vi "SQLite Add Saving Goal Test.vi"(7 "Test DB Set Up Command":string, 8 "Error In (no error)":errorcluster, 11 "SQLite DB Operator In":refnum<class "SQLite DB Operator.lvclass">) -> (0 "Error Out":errorcluster, 3 "SQLite DB Operator Out":refnum<class "SQLite DB Operator.lvclass">)   [LabVIEW 2023]
uses:
  Clasess/SQLite DB Operator/SQLite DB Operator.lvclass
  Clasess/DB Records/Expenses Tracker Saving Goal/Public/Ctrls/Saving Goal.ctl
  Clasess/DB Records/Expenses Tracker Saving Goal/Expenses Tracker Saving Goal.lvclass
  H:/Desktop/LabVIEW/LabView Repo/Expenses-Tracker-DB-Operator/Interfaces/Expenses Tracker Record/Expenses Tracker Record.lvclass
  Clasess/DB Records/Expenses Tracker Transaction/Expenses Tracker Transaction.lvclass
  Support/Adding/Add Record Assert Error.vi
  Support/Adding/Add Record Assert Not Error.vi
  <vilib>/drjdpowell/SQLite Library/SQL Connection/Execute SQL (1D Cluster).vi
  <vilib>/addons/_JKI Toolkits/Caraya/classes/Test/Test.lvclass
  <vilib>/drjdpowell/SQLite Library/SQLite.lvlib
  H:/Desktop/LabVIEW/LabView Repo/Expenses-Tracker-DB-Operator/Clasess/DB Records/Expenses Tracker Saving Goal/Expenses Tracker Saving Goal.lvclass
  <vilib>/drjdpowell/SQLite Library/SQL Connection/Connection.lvclass
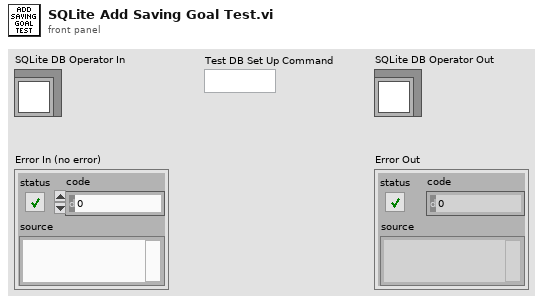
[diagram p1: front panel]
types:
  T1 = typedef "Expenses Tracker Saving Goal.lvclass/Saving Goal.ctl" = cluster{"ID":u32, "Name":string, "Current_value":dbl, "Target_value":dbl, "Date_of_entry":timestamp, "Due_date":timestamp, "Last_update":timestamp, "Description":string}
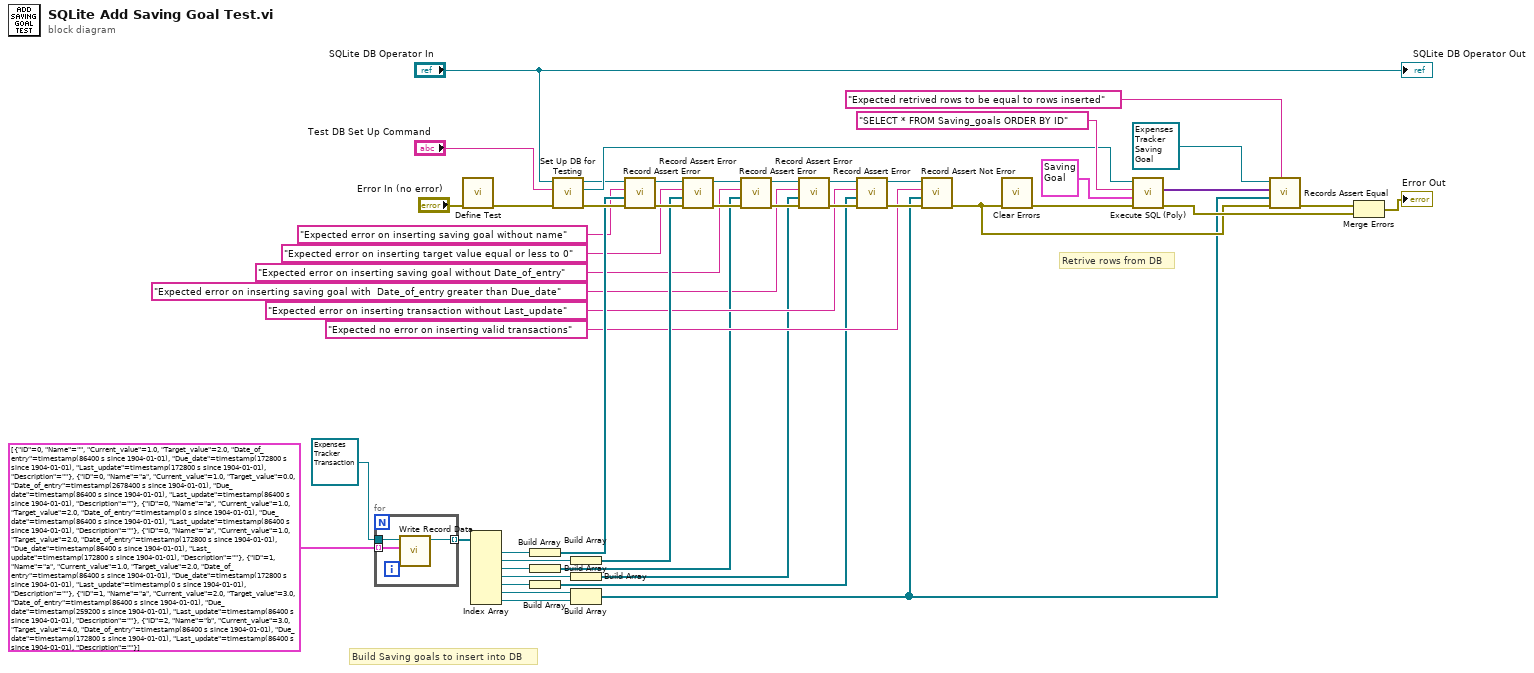
[diagram p0: block diagram]
diagram:
  (unwired) refnum<class "Expenses Tracker Transaction.lvclass"> refnum ("Expenses Tracker Category")
  # "Retrive rows from DB"
  # "Build Saving goals to insert into DB"
  n1 = for {
    tunnel: T1[] [{"ID"=0, "Name"="", "Current_value"=1.0, "Target_value"=2.0, "Date_of_entry"=timestamp(86400 s since 1904-01-01), "Due_date"=timestamp(172800 s since 1904-01-01), "Last_update"=timestamp(172800 s since 1904-01-01), "Description"=""}, {"ID"=0, "Name"="a", "Current_value"=1.0, "Target_value"=0.0, "Date_of_entry"=timestamp(2678400 s since 1904-01-01), "Due_date"=timestamp(86400 s since 1904-01-01), "Last_update"=timestamp(86400 s since 1904-01-01), "Description"=""}, {"ID"=0, "Name"="a", "Current_value"=1.0, "Target_value"=2.0, "Date_of_entry"=timestamp(0 s since 1904-01-01), "Due_date"=timestamp(86400 s since 1904-01-01), "Last_update"=timestamp(86400 s since 1904-01-01), "Description"=""}, {"ID"=0, "Name"="a", "Current_value"=1.0, "Target_value"=2.0, "Date_of_entry"=timestamp(172800 s since 1904-01-01), "Due_date"=timestamp(86400 s since 1904-01-01), "Last_update"=timestamp(172800 s since 1904-01-01), "Description"=""}, {"ID"=1, "Name"="a", "Current_value"=1.0, "Target_value"=2.0, "Date_of_entry"=timestamp(86400 s since 1904-01-01), "Due_date"=timestamp(172800 s since 1904-01-01), "Last_update"=timestamp(0 s since 1904-01-01), "Description"=""}, {"ID"=1, "Name"="a", "Current_value"=2.0, "Target_value"=3.0, "Date_of_entry"=timestamp(86400 s since 1904-01-01), "Due_date"=timestamp(259200 s since 1904-01-01), "Last_update"=timestamp(86400 s since 1904-01-01), "Description"=""}, {"ID"=2, "Name"="b", "Current_value"=3.0, "Target_value"=4.0, "Date_of_entry"=timestamp(86400 s since 1904-01-01), "Due_date"=timestamp(172800 s since 1904-01-01), "Last_update"=timestamp(86400 s since 1904-01-01), "Description"=""}] ("Array") -> [w52] mode=indexing
    tunnel: refnum<class "Expenses Tracker Saving Goal.lvclass"> refnum ("Expenses Tracker Category") -> [w50]
    tunnel: [w51] -> w47 mode=indexing
    n2 = call-dynamic "Write Record Data.vi"("Record"=w52, "Expenses Tracker Saving Goal In"=w50) -> ("Expenses Tracker Saving Goal Out"=w51:refnum<class "Expenses Tracker Saving Goal.lvclass">)  [unwired: 8 in, 1 out]
  }
  n3 = call <vilib>:"Define Test.vi"("error in (no error)"="Error In (no error)") -> ("error out"=w41:errorcluster)  [unwired: 9 in, 1 out]
  n4 = Index Array(array=w47) -> (element #1=w23:refnum<class "Expenses Tracker Saving Goal.lvclass">, element #2=w19:refnum<class "Expenses Tracker Saving Goal.lvclass">, element #3=w14:refnum<class "Expenses Tracker Saving Goal.lvclass">, element #4=w12:refnum<class "Expenses Tracker Saving Goal.lvclass">, element #5=w10:refnum<class "Expenses Tracker Saving Goal.lvclass">, element #6=w2:refnum<class "Expenses Tracker Saving Goal.lvclass">, element #7=w1:refnum<class "Expenses Tracker Saving Goal.lvclass">)  [unwired: 7 in]
  n5 = Build Array(w23) -> (w22:refnum<class "Expenses Tracker Saving Goal.lvclass">[])
  n6 = Build Array(w14) -> (w13:refnum<class "Expenses Tracker Saving Goal.lvclass">[])
  n7 = Build Array(w10) -> (w9:refnum<class "Expenses Tracker Saving Goal.lvclass">[])
  n8 = call "Set Up DB for Testing.vi"("Error In (no error)"=w41, "Test DB Set Up Command"="Test DB Set Up Command", "SQLite DB Operator In"="SQLite DB Operator In") -> ("Error Out"=w25:errorcluster, "SQLite Connection"=w44:refnum<class "Connection.lvclass">, "SQLite DB Operator Out"=w21:refnum<class "SQLite DB Operator.lvclass">)  [unwired: 6 in]
  n9 = Build Array(w19) -> (w18:refnum<class "Expenses Tracker Saving Goal.lvclass">[])
  n10 = Build Array(w12) -> (w11:refnum<class "Expenses Tracker Saving Goal.lvclass">[])
  n11 = Build Array(w2, w1) -> (w3:refnum<class "Expenses Tracker Saving Goal.lvclass">[])
  n12 = call-poly "Record Assert Error.vi"("Error In"=w25, "Records"=w22, "Assertion Label"="Expected error on inserting saving goal without name" ("Label (VI Title)"), "SQLite DB Operator In"=w21) -> ("Error Out"=w32:errorcluster, "SQLite DB Operator Out"=w33:refnum<class "SQLite DB Operator.lvclass">)  [unwired: 6 in]
  n13 = call-poly "Record Assert Error.vi"("Error In"=w32, "Records"=w18, "Assertion Label"="Expected error on inserting target value equal or less to 0" ("Label (VI Title)"), "SQLite DB Operator In"=w33) -> ("Error Out"=w30:errorcluster, "SQLite DB Operator Out"=w31:refnum<class "SQLite DB Operator.lvclass">)  [unwired: 6 in]
  n14 = call-poly "Record Assert Error.vi"("Error In"=w30, "Records"=w13, "Assertion Label"="Expected error on inserting saving goal without Date_of_entry" ("Label (VI Title)"), "SQLite DB Operator In"=w31) -> ("Error Out"=w35:errorcluster, "SQLite DB Operator Out"=w34:refnum<class "SQLite DB Operator.lvclass">)  [unwired: 6 in]
  n15 = call-poly "Record Assert Error.vi"("Error In"=w35, "Records"=w11, "Assertion Label"="Expected error on inserting saving goal with  Date_of_entry greater than Due_date" ("Label (VI Title)"), "SQLite DB Operator In"=w34) -> ("Error Out"=w28:errorcluster, "SQLite DB Operator Out"=w29:refnum<class "SQLite DB Operator.lvclass">)  [unwired: 6 in]
  n16 = call-poly "Record Assert Error.vi"("Error In"=w28, "Records"=w9, "Assertion Label"="Expected error on inserting transaction without Last_update" ("Label (VI Title)"), "SQLite DB Operator In"=w29) -> ("Error Out"=w26:errorcluster, "SQLite DB Operator Out"=w27:refnum<class "SQLite DB Operator.lvclass">)  [unwired: 6 in]
  n17 = call-poly "Record Assert Not Error.vi"("Error In"=w26, "Records"=w3, "Assertion Label"="Expected no error on inserting valid transactions" ("Label (VI Title)"), "SQLite DB Operator In"=w27) -> ("Error Out"=w24:errorcluster)  [unwired: 6 in, 1 out]
  n18 = call <vilib>:"Clear Errors.vi"("error in (no error)"=w24) -> ("error out"=w36:errorcluster)  [unwired: 5 in, 1 out]
  n19 = call-poly <vilib>:"Execute SQL (Poly).vi"("error in (no error)"=w36, "Cluster (or Array of Clusters)"=T1 {"ID"=0, "Name"="", "Current_value"=0.0, "Target_value"=0.0, "Date_of_entry"=timestamp(0 s since 1904-01-01), "Due_date"=timestamp(0 s since 1904-01-01), "Last_update"=timestamp(0 s since 1904-01-01), "Description"=""} ("Saving Goal"), "SQL"="SELECT * FROM Saving_goals ORDER BY ID", "SQLite Connection in"=w44) -> ("error out"=w37:errorcluster, "Result Set (Array of Clusters)"=w8:variant[])  [unwired: 5 in, 1 out]
  n20 = call "Records Assert Equal.vi"("Assertion Label"="Expected retrived rows to be equal to rows inserted" ("Label (VI Title)"), "Error In"=w24, "Correct Records"=w3, "Typedef Records"=w8, "Expenses Tracker Record In"=refnum<class "Expenses Tracker Saving Goal.lvclass"> refnum ("Expenses Tracker Category")) -> ("Error Out"=w38:errorcluster)  [unwired: 6 in]
  n21 = Merge Errors(w38, w37) -> (→"Error Out":errorcluster)
  "SQLite DB Operator Out" <- "SQLite DB Operator In"
